vi "set Header.vi"(10 "Header":string, 11 "Log.lvclass in":refnum<class "Log.lvclass">) -> (3 "Log.lvclass out":refnum<class "Log.lvclass">)   [LabVIEW 2020, in "Log.lvclass"]
uses:
  Log.lvclass
  Log.lvclass/Log.ctl
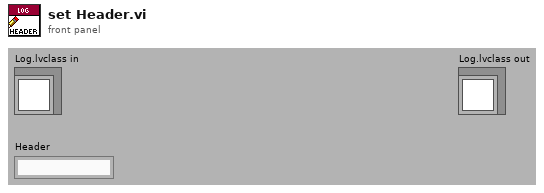
[diagram p1: front panel]
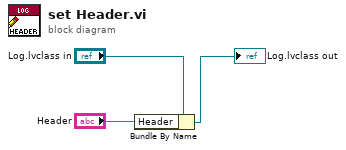
[diagram p0: block diagram]
diagram:
  n1 = Bundle By Name(cluster="Log.lvclass in", "Header"="Header") -> (→"Log.lvclass out":refnum<class "Log.lvclass">)
